vi "PCert-ConfigPageNF-InitializeActorToDBCC.vi"(7 "JSON String":string, 8 "error in (no error)":errorcluster, 11 "ERP-ConfigPageNF in":refnum<class "PCert-ConfigPageNF.lvclass">) -> (0 "error out":errorcluster, 1 "Actor PageID":string, 2 "Plugin Caller Ref":refnum<class "FTW-ActorConnector.lvclass">, 3 "ERP-ConfigPageNF out":refnum<class "PCert-ConfigPageNF.lvclass">)   [LabVIEW 2013, in "PCert-ConfigPageNF.lvclass"]
uses:
  PCert-ConfigPageNF.lvclass
  ftw-dataflow/Actor/src/Connector/FTW-ActorConnector.lvclass
  PCert-ConfigPageNF.lvclass/PCert-ConfigPageNF.ctl
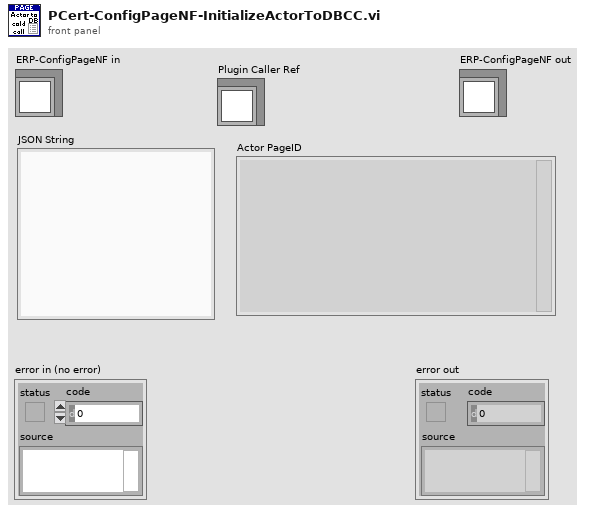
[diagram p1: front panel]
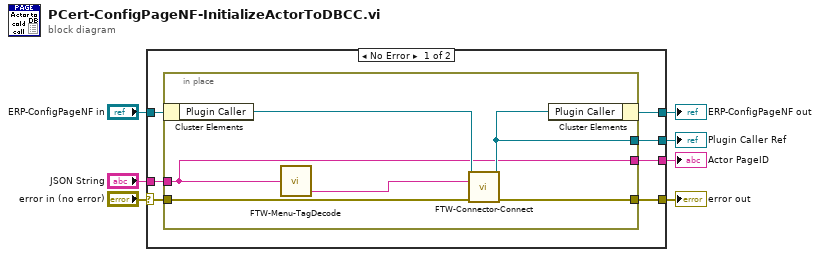
[diagram p0: block diagram]
diagram:
  n1 = case shown="No Error" "error in (no error)" {
    selector: "error in (no error)" -> [w14 w22]
    tunnel: [w12 w22] -> w6
    tunnel: [w10 w21] -> w4
    tunnel: "ERP-ConfigPageNF in" -> [w11 w21]
    tunnel: "JSON String" -> [w13 _]
    tunnel: [w9 _] -> w2
    tunnel: [w8 _] -> w1
    frame No Error {
      n2 = in-place {
        in-place-border: w14 -> [w17]
        in-place-border: w13 -> [w15]
        in-place-border: [w19] -> w12
        in-place-border: [w15] -> w9
        in-place-border: [w18] -> w8
        n3 = in-place-cluster #1(w11) -> ("Plugin Caller"=w20:refnum<class "FTW-ActorConnector.lvclass">)
        n4 = call "FTW-Menu-TagDecode.vi"("Menu Item Tag"=w15) -> ("Payload"=w16:string)  [unwired: 3 out]
        n5 = call-dynamic "FTW-Connector-Connect.vi"("FTW Actor Connector Type"=w20, "Instance Inbox Address"=w16, "error in"=w17) -> ("FTW Actor Connector"=w18:refnum<class "FTW-ActorConnector.lvclass">, "error out"=w19:errorcluster)  [unwired: 11 in]
        n6 = in-place-cluster #1("Plugin Caller"=w18) -> (w10:refnum<class "PCert-ConfigPageNF.lvclass">)
      }
    }
    frame Error {
    }
  }
  "error out" <- w6
  "ERP-ConfigPageNF out" <- w4
  "Actor PageID" <- w2
  "Plugin Caller Ref" <- w1
